vi "LED Control Module Main.vi"() -> ()   [LabVIEW 2018, in "LED Control Module.lvlib"]
uses:
  LED Control Module.lvlib
  Public Controls/LVS Settings.ctl
  Public Controls/LVS Limits.ctl
  Public Controls/LVS Instruments.ctl
  Modules/Entry Console/Entry Console/Public Controls/Entry Console.ctl
  Public Controls/TestData.ctl
  INI/INI File Control.ctl
  Public Controls/LVS Testplan.ctl
  Private Controls/Module Data Cluster.ctl
  Private Controls/Module Action.ctl
  <vilib>/Utility/error.llb/DialogType.ctl
  User Events/controls/Actions.ctl
  Modules/Display Console/Display Console/public controls/Display Data.ctl
  Modules/Entry Console/Entry Console/Public Controls/Button Status.ctl
  Modules/Display Console/Display Console/Display.lvlib
  Modules/Entry Console/Entry Console/Entry Console.lvlib
  INI/LED INI File.lvlib
panel:
  in  "LED Validation":enum32{"Validation", "Settings"}(tab)
  out "Test Visualize":cluster{dbl[], dbl[]}[](graph)=[{[0.0, 0.0, 0.0], [0.0, nan, nan]}, {[-0.05, 0.0], [0.0, 0.0]}, {[-0.05, 0.0], [0.0, 0.0]}] caption="LED Current Consumption"
  out "Messages":string
  in  "History":i32(listbox)
  in  "Tester Status":string
  out "Test Status":bool=TRUE
  out "Instruments":T1 caption="LED Reference Resistors" {"Resistor 3" format="%#_g ohm"; "Resistor 2" format="%#_g ohm"; "Resistor 1" format="%#f ohm"}
  in  "Exit":bool
  in  "Logout":bool
  out "Part Number":string
  in  "Test Control":bool
  in  "Clear":bool
  out "LED":bool
  out "Settings":T2 {"Source V" format="%#_g V"; "VLED 3" format="%#_g V"; "VLED 2" format="%#_g V"; "VLED 1" format="%#f V"}
  out "Limits":T3 {"Wavelength" format="%#_g nm"; "Tolerance" format="%#_g %"; "Current 3" format="%#_g  mA"; "Current 2" format="%#_g  mA"; "Current 1" format="%#_g mA"}
  in  "Role":string
  in  "Username":string
  out "error out":errorcluster
  in  "error in":errorcluster
  # "LED Validation SYsTEM"
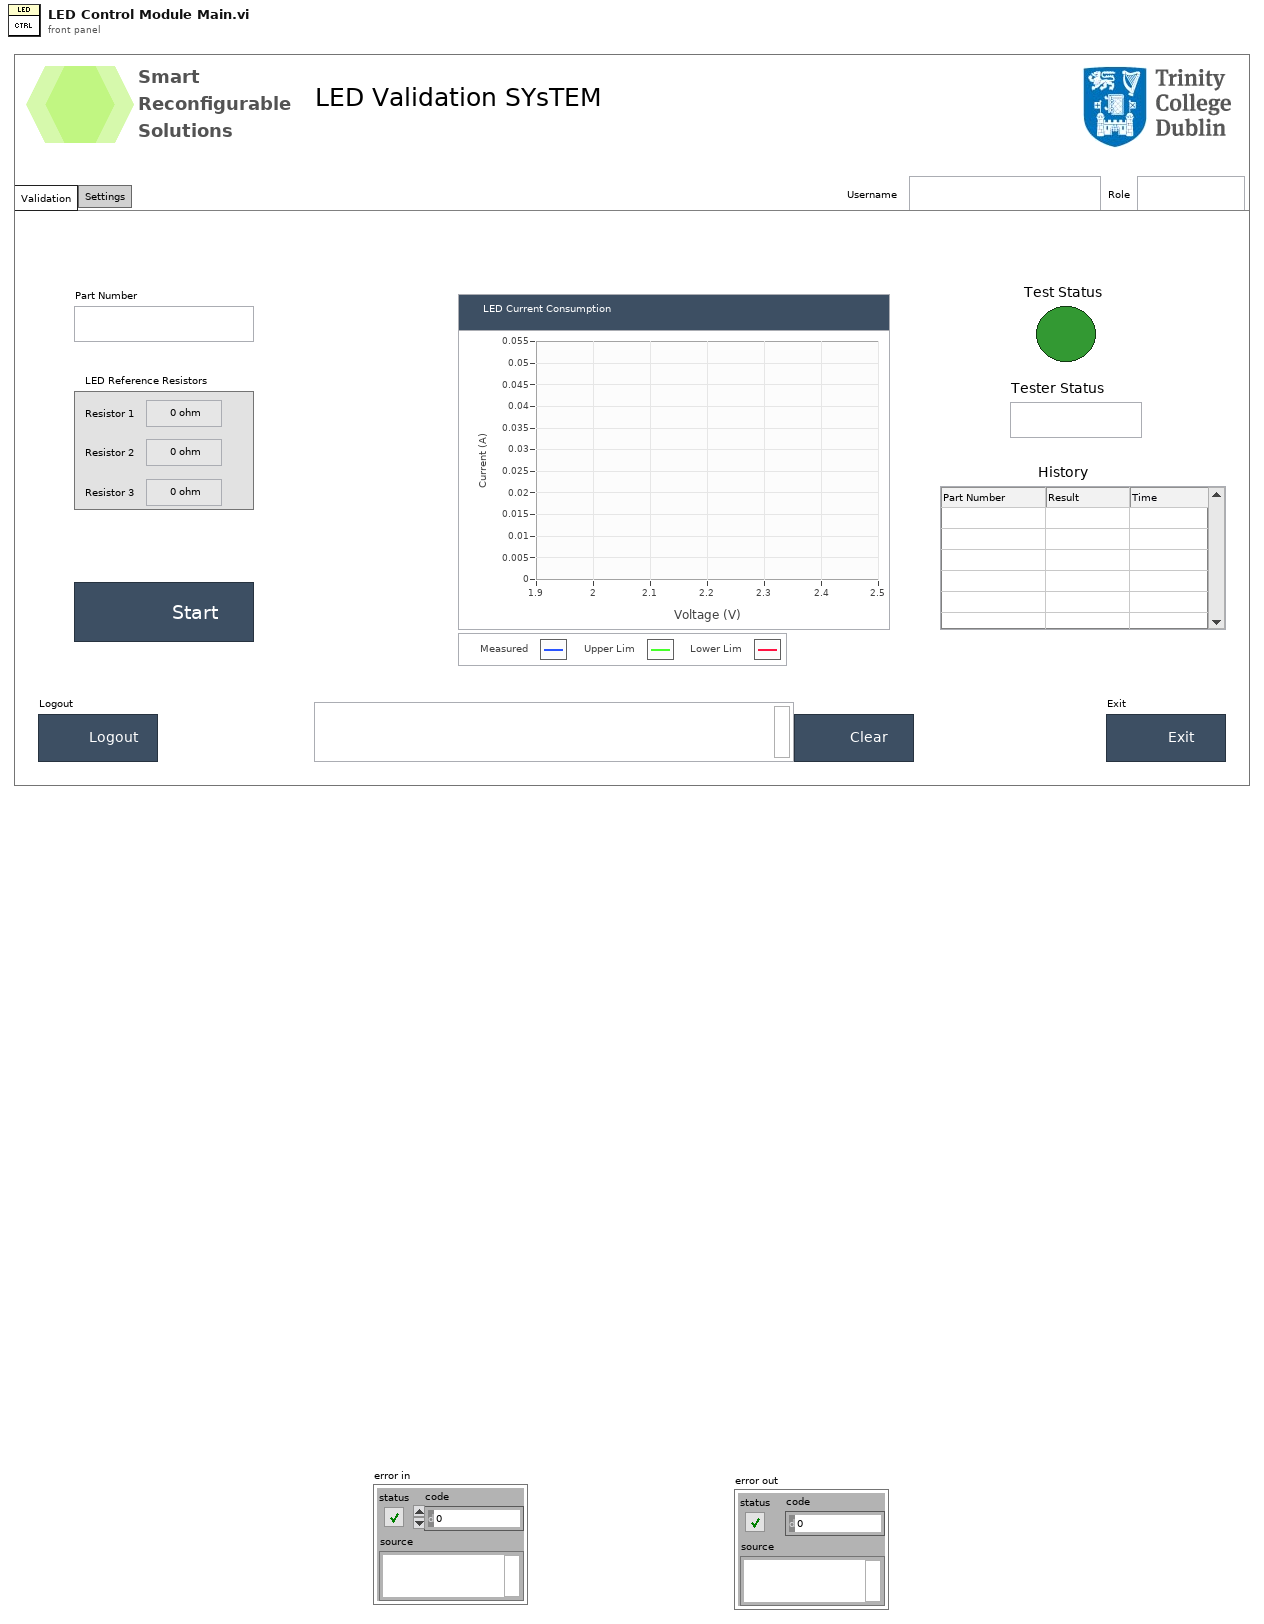
[diagram p1: front panel]
types:
  T1 = typedef "LED Control Module.lvlib/LVS Instruments.ctl" = cluster{"Resistor 1":dbl, "Resistor 2":dbl, "Resistor 3":dbl}
  T2 = typedef "LED Control Module.lvlib/LVS Settings.ctl" = cluster{"VLED 1":dbl, "VLED 2":dbl, "VLED 3":dbl, "Source V":dbl}
  T3 = typedef "LED Control Module.lvlib/LVS Limits.ctl" = cluster{"Current 1":dbl, "Current 2":dbl, "Current 3":dbl, "Tolerance":dbl, "Wavelength":dbl}
  T4 = typedef "LED Control Module.lvlib/TestData.ctl" = cluster{"data":T5, "Result Cluster":cluster{"TestResult":T6, "full date string":string, "Result":bool, "Part Number":string}}
  T5 = typedef "LED Control Module.lvlib/LED INI File.lvlib/INI File Control.ctl" = cluster{"TestPlan":T6, "Instruments":T1, "Limits":T3, "Settings":T2}
  T6 = typedef "LED Control Module.lvlib/LVS Testplan.ctl" = cluster{"Current Consumption":bool, "Emission Spectrum":bool}
  T7 = typedef "Entry Console.lvlib/Entry Console.ctl" = cluster{"Variant":variant}
  T8 = cluster{"Step Duration":string, "Station":string, "Wash Step":string}[]
  T9 = typedef "Actions.ctl" = enum16{"Get", "Create", "Destroy"}
  T10 = typedef "Display.lvlib/Display Data.ctl" = cluster{"Variant":variant}
  T11 = typedef "LED Control Module.lvlib/Module Data Cluster.ctl" = cluster{"Variant":variant, "action":T12}
  T12 = typedef "LED Control Module.lvlib/Module Action.ctl" = enum16{"exit", "error", "init", "close", "start", "Current", "Spectrum", "WriteResult"}
  T13 = typedef "DialogType.ctl" = u16
  T14 = typedef "Entry Console.lvlib/Button Status.ctl" = cluster{"Enable  ctrl1":bool, "reset":bool, "Enable ctrl2":bool}
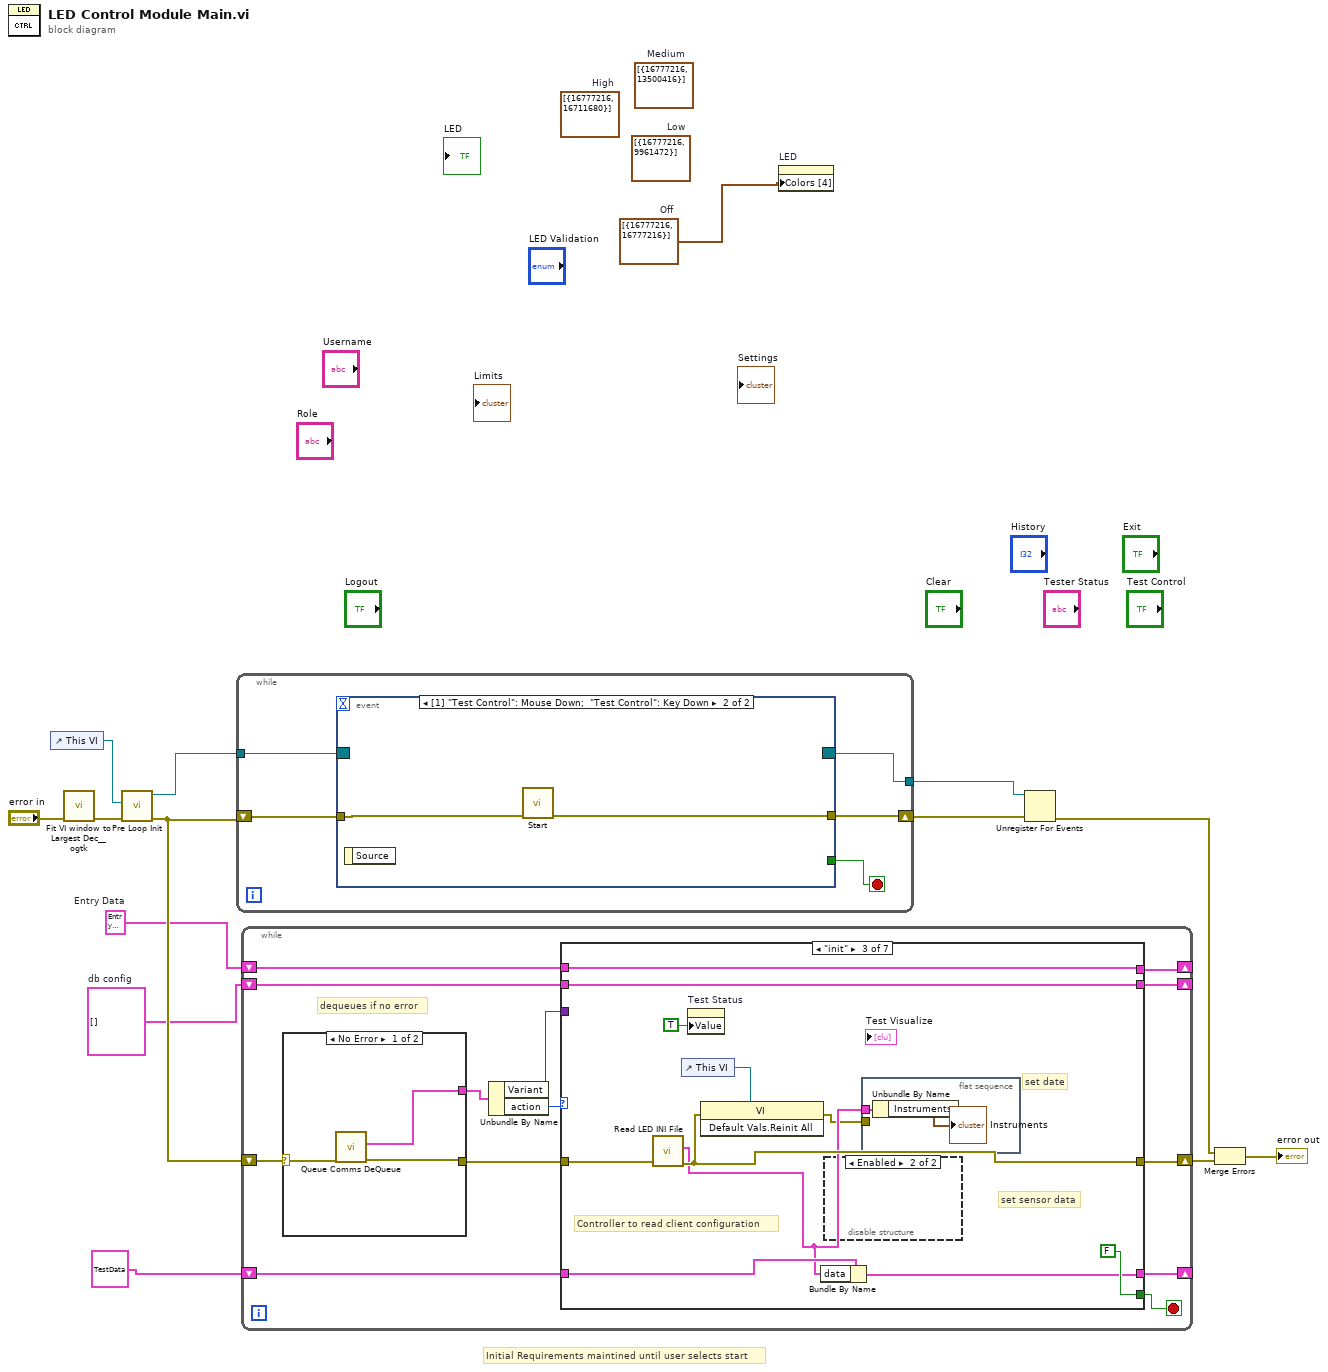
[diagram p0: block diagram]
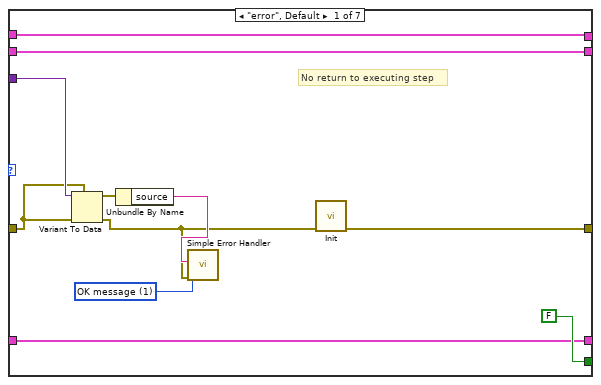
[diagram p2: hidden frame]
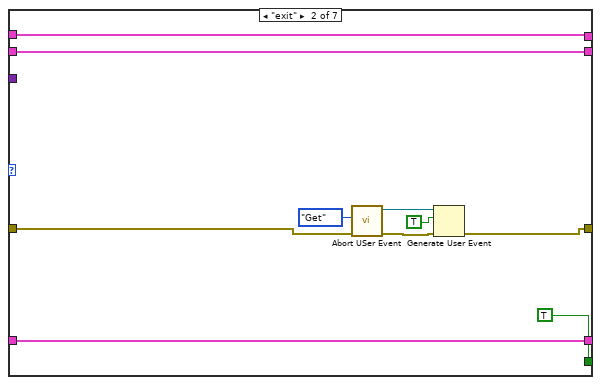
[diagram p3: hidden frame]
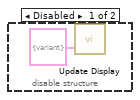
[diagram p4: hidden frame]
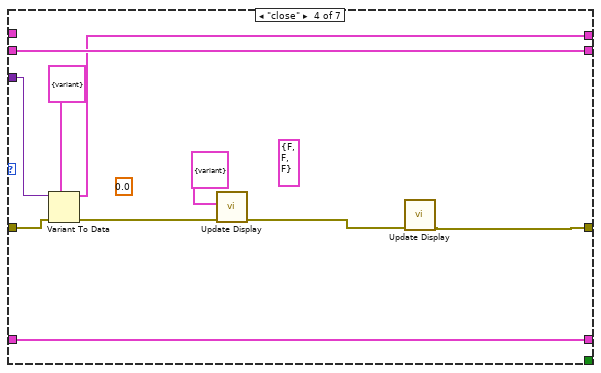
[diagram p5: hidden frame]
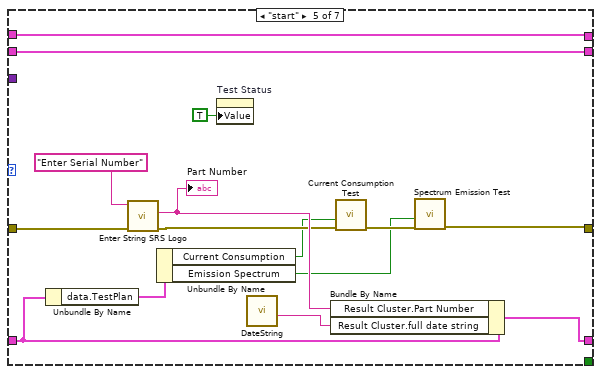
[diagram p6: hidden frame]
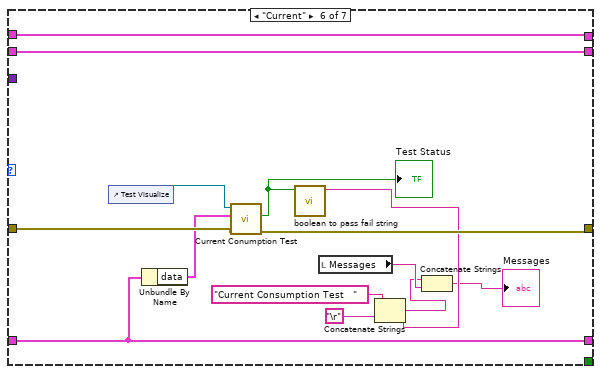
[diagram p7: hidden frame]
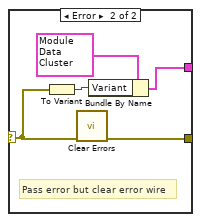
[diagram p9: hidden frame]
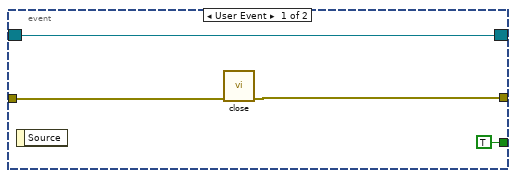
[diagram p10: hidden frame]
diagram:
  w2 = cluster{u32, u32}[] [{16777216, 16777216}]  # Off
  (unwired) cluster{u32, u32}[] [{16777216, 9961472}]  # Low
  (unwired) cluster{u32, u32}[] [{16777216, 13500416}]  # Medium
  (unwired) cluster{u32, u32}[] [{16777216, 16711680}]  # High
  w6 = T7 {"Variant"=variant}  # Entry Data
  w5 = T8 []  # db config
  # "Initial Requirements maintined until user selects start"
  n1 = control-ref of="This VI"() -> (w14:refnum<vi>)
  n2 = call <userlib>:"Fit VI window to Largest Dec__ogtk.vi"("error in (no error)"="error in") -> ("error out"=w3:errorcluster)  [unwired: 5 in, 1 out]
  n3 = call "Pre Loop Init.vi"("error in"=w3, "Ref In"=w14) -> ("error out"=w12:errorcluster, "Event Registration Refnum"=w13:refnum<event-registration>)  [unwired: 8 in]
  n4 = while {
    shift-right: [w18] -> w11
    shift-left: w12 -> [w19]
    tunnel: w13 -> [w17]
    tunnel: [w15] -> w10
    stop <- w16 stop-if-true
    n5 = event shown="[1] \"Test Control\": Mouse Down;  \"Test Control\": Key Down" {
      selector: w17 -> [w20 _]
      dyn-events: [w20 _] -> w15
      timeout: _ -> [_ _]
      tunnel: w19 -> [w23 w25]
      tunnel: [w22 w24] -> w18
      tunnel: [TRUE _] -> w16
      event User Event {
        n6 = event-data() -> ()  [unwired: 1 in, 1 out]
        n7 = call "close.vi"("error in"=w23) -> ("error out"=w22:errorcluster)  [unwired: 10 in]
      }
      event "Test Control": Mouse Down; "Test Control": Key Down {
        n8 = event-data() -> ()  [unwired: 1 in, 1 out]
        n9 = call "Start.vi"("error in"=w25) -> ("error out"=w24:errorcluster)  [unwired: 10 in]
      }
    }
  }
  n10 = while {
    shift-right: [w35] -> w9
    shift-left: w12 -> [w38]
    shift-right: [w32] -> _
    shift-left: w5 -> [w31]
    shift-right: [w30] -> _
    shift-left: w6 -> [w29]
    shift-right: [w26] -> _
    shift-left: T4 {"data"={"TestPlan"={"Current Consumption"=TRUE, "Emission Spectrum"=TRUE}, "Instruments"={"Resistor 1"=0.0, "Resistor 2"=0.0, "Resistor 3"=0.0}, "Limits"={"Current 1"=0.0, "Current 2"=0.0, "Current 3"=0.0, "Tolerance"=0.0, "Wavelength"=0.0}, "Settings"={"VLED 1"=0.0, "VLED 2"=0.0, "VLED 3"=0.0, "Source V"=0.0}}, "Result Cluster"={"TestResult"={"Current Consumption"=FALSE, "Emission Spectrum"=FALSE}, "full date string"="", "Result"=FALSE, "Part Number"=""}} ("TestData") -> [w27]
    stop <- w33 stop-if-true
    # "dequeues if no error"
    n11 = case shown="No Error" w38 {
      selector: w38 -> [w119 w124]
      tunnel: [w118 w120] -> w37
      tunnel: [w117 w123] -> w34
      frame No Error {
        n12 = call "Queue Comms DeQueue.vi"("error in"=w119) -> ("error out"=w117:errorcluster, "element"=w118:T11)  [unwired: 9 in]
      }
      frame Error {
        # "Pass error but clear error wire"
        n13 = To Variant(anything=w124) -> (Variant=w121:variant)
        n14 = call <vilib>:"Clear Errors.vi"("error in (no error)"=w124) -> ("error out"=w123:errorcluster)  [unwired: 5 in, 1 out]
        n15 = Bundle By Name(cluster=T11 {"Variant"=variant, "action"=enum."error"} ("element"), "Variant"=w121) -> (w120:T11)
      }
    }
    n16 = Unbundle By Name(w37) -> ("Variant"=w36:variant, "action"=w28:T12)
    n17 = case shown="\"init\"" w28 {
      tunnel: w36 -> [w45 _ _ w81 _ _ _]
      tunnel: [w41 w51 w65 w77 w88 w109 w116] -> w35
      tunnel: w34 -> [w44 w52 w67 w79 w95 w110 w116]
      tunnel: [FALSE TRUE FALSE _ _ _ _] -> w33
      tunnel: [w48 w58 w69 w82 w98 w112 w115] -> w32
      tunnel: w31 -> [w48 w58 w69 w82 w98 w112 w115]
      tunnel: [w47 w57 w68 w78 w97 w111 w114] -> w30
      tunnel: w29 -> [w47 w57 w68 _ w97 w111 w114]
      tunnel: w27 -> [w39 w50 w64 w74 w92 w108 w113]
      tunnel: [w39 w50 w63 w74 w94 w108 w113] -> w26
      frame "error", Default {
        w46 = T13 1 items=["no dialog", "OK message", "continue or stop message", "OK message + warnings", "continue/stop + warnings"] ("type of dialog (OK msg:1)")
        # "No return to executing step"
        n18 = Variant To Data(error in=w44, type=w44, Variant=w45) -> (data=w43:errorcluster, error out=w40:errorcluster)
        n19 = Unbundle By Name(w43) -> ("source"=w42:string)
        n20 = call <vilib>:"Simple Error Handler.vi"("error source (\" \")"=w42, "type of dialog (OK msg:1)"=w46, "error in (no error)"=w40) -> ()  [unwired: 2 in, 5 out]
        n21 = call "Init.vi"("error in"=w40) -> ("error out"=w41:errorcluster)  [unwired: 10 in]
      }
      frame "exit" {
        n22 = call "Abort USer Event.vi"("error in"=w52, "Enum"=Actions."Get") -> ("error out"=w54:errorcluster, "user event out"=w53:refnum<user-event>)  [unwired: 8 in]
        n23 = Generate User Event(user event=w53, event data cluster=TRUE ("event data"), error in=w54) -> (error out=w51:errorcluster)  [unwired: 1 in, 1 out]
      }
      frame "init" {
        # "set sensor data"
        # "set date"
        # "Controller to read client configuration"
        n24 = call "Read LED INI File.vi"("error in"=w67) -> ("error out"=w65:errorcluster, "data"=w61:T5)  [unwired: 9 in]
        n25 = control-ref of="This VI"() -> (w66:refnum<vi>)
        n26 = property on="Test Status" class="Bool (strict)"("Value"=TRUE ("Test Status")) -> ()  [unwired: 2 in, 2 out]
        n27 = invoke class="VI" method="Default Vals.Reinit All"(reference=w66, error in=w65) -> (error out=w60:errorcluster)  [unwired: 1 in, 2 out]
        n28 = Bundle By Name(cluster=w64, "data"=w61) -> (w63:T4)
        n29 = disable-structure shown="Enabled" {
          frame Disabled {
            n30 = call "Update Display.vi"("data"=T10 {"Variant"=variant(cluster{"Variant":variant} {"Variant"=variant})} ("Cluster")) -> ()  [unwired: 10 in, 1 out]
          }
          frame Enabled {
          }
        }
        n31 = flat-sequence {
          tunnel: w61 -> [w72]
          tunnel: w60 -> [_]
          frame #0 {
            n32 = Unbundle By Name(w72) -> ("Instruments"=→"Instruments":T1)
          }
        }
      }
      frame "close" {
        (unwired) 0.0
        (unwired) T14 {"Enable  ctrl1"=FALSE, "reset"=FALSE, "Enable ctrl2"=FALSE}
        n33 = Variant To Data(error in=w79, type=T7 {"Variant"=variant} ("WashStepSelection"), Variant=w81) -> (data=w78:T7, error out=w76:errorcluster)
        n34 = call "Update Display.vi"("error in"=w76, "data"=T10 {"Variant"=variant} ("Cluster")) -> ("error out"=w75:errorcluster)  [unwired: 9 in]
        n35 = call "Update Display.vi"("error in"=w75) -> ("error out"=w77:errorcluster)  [unwired: 10 in]
      }
      frame "start" {
        n36 = Unbundle By Name(w92) -> ("data.TestPlan"=w91:T6)
        n37 = call "Enter String SRS Logo.vi"("error in"=w95, "Message"="Enter Serial Number") -> ("error out"=w90:errorcluster, "String Value"=w93:string)  [unwired: 8 in]
        "Part Number" <- w93
        n38 = Unbundle By Name(w91) -> ("Current Consumption"=w87:bool, "Emission Spectrum"=w86:bool)
        n39 = property on="Test Status" class="Bool (strict)"("Value"=TRUE ("Test Status")) -> ()  [unwired: 2 in, 2 out]
        n40 = call "DateString.vi"() -> ("full date string"=w85:string)  [unwired: 7 in, 4 out]
        n41 = Bundle By Name(cluster=w92, "Result Cluster.Part Number"=w93, "Result Cluster.full date string"=w85) -> (w94:T4)
        n42 = call "Current Consumption Test.vi"("error in"=w90, "Execute"=w87) -> ("error out"=w89:errorcluster)  [unwired: 9 in]
        n43 = call "Spectrum Emission Test.vi"("error in"=w89, "Execute"=w86) -> ("error out"=w88:errorcluster)  [unwired: 9 in]
      }
      frame "Current" {
        n44 = control-ref of="Test Visualize"() -> (w106:refnum<vi>)
        n45 = Unbundle By Name(w108) -> ("data"=w107:T5)
        n46 = call "Current Conumption Test.vi"("error in"=w110, "LED INI"=w107, "Test Visualize In"=w106) -> ("error out"=w109:errorcluster, "Pass Fail"=w104:bool)  [unwired: 6 in, 1 out]
        "Test Status" <- w104
        n47 = call "boolean to pass fail string.vi"("Boolean"=w104) -> ("Stat"=w103:string)  [unwired: 9 in, 1 out]
        n48 = local read "Messages"() -> (w105:string)
        n49 = Concatenate Strings("Current Consumption Test   " ("String Control"), w103, "\r") -> (w101:string)
        n50 = Concatenate Strings(w101, w105) -> (→"Messages":string)
      }
      frame "Spectrum" {
      }
    }
  }
  n51 = property on="LED" class="Bool (strict)"("Colors [4]"=w2) -> ()  [unwired: 2 in, 2 out]
  n52 = Unregister For Events(event registration refnum=w10, error in=w11) -> (error out=w7:errorcluster)
  n53 = Merge Errors(w7, w9) -> (→"error out":errorcluster)
